vi "DAQmx PWM PID.vi"(9 "PID gains":T1={"proportional gain (Kc)"=1.0, "integral time (Ti, min)"=0.01, "derivative time (Td, min)"=0.0}, 10 "Process Variable":dbl, 11 "Setpoint":dbl) -> (0 "Control Output":dbl)   [LabVIEW 2023]
uses:
  <vilib>/addons/control/pid/pid.llb/PID (DBL).vi
  <vilib>/addons/control/pid/NI_PID_pid.lvlib
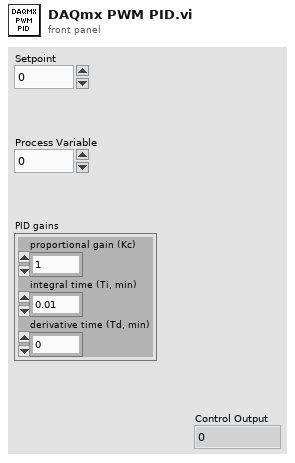
[diagram p1: front panel]
types:
  T1 = cluster{"proportional gain (Kc)":dbl, "integral time (Ti, min)":dbl, "derivative time (Td, min)":dbl}
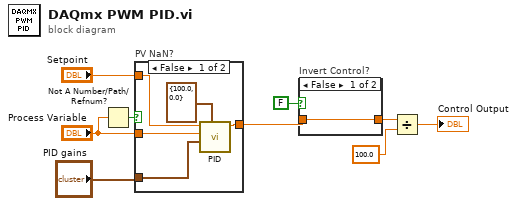
[diagram p0: block diagram]
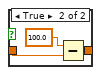
[diagram p2: hidden frame]
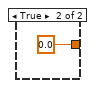
[diagram p3: hidden frame]
diagram:
  n1 = Not A Number/Path/Refnum?(number/path/refnum="Process Variable") -> (NaN/Path/Refnum?=w7:bool)
  n2 = case "PV NaN?" shown="False" w7 {
    tunnel: "Setpoint" -> [w13 _]
    tunnel: [w12 0.0 ("output")] -> w6
    tunnel: "Process Variable" -> [w11 _]
    tunnel: "PID gains" -> [w10 _]
    frame False {
      n3 = call-poly <vilib>:"PID.vi"("output range"=cluster{"output high":dbl, "output low":dbl} {"output high"=100.0, "output low"=0.0}, "PID gains"=w10, "process variable"=w11, "setpoint"=w13) -> ("output"=w12:dbl)  [unwired: 6 in, 1 out]
    }
    frame True {
    }
  }
  n4 = case "Invert Control?" shown="False" FALSE {
    tunnel: w6 -> [w16 w19]
    tunnel: [w16 w18] -> w3
    frame False {
    }
    frame True {
      n5 = Subtract(x=100.0, y=w19) -> (x-y=w18:dbl)
    }
  }
  n6 = Divide(x=w3, y=100.0) -> (x/y=→"Control Output":dbl)
